vi "PXI-Set AO Gains and Multipliers.vi"(0 "Multipliers":dbl[](array[numeric]), 5 "Gains":dbl[](array[numeric]), 7 "AO Channels":i32[](array[numeric]), 11 "error in (no error)":errorcluster) -> (15 "error out":errorcluster)   [LabVIEW 2020]
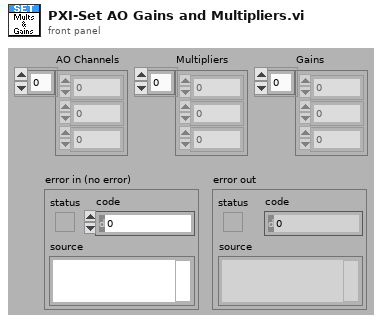
[diagram p1: front panel]
types:
  T1 = enum16{"Init", "Write", "Read", "Latch setup", "Compute comp."}
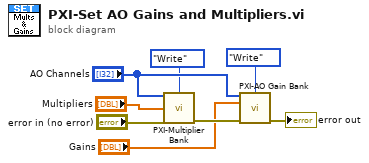
[diagram p0: block diagram]
diagram:
  n1 = call "PXI-Multiplier Bank.vi"("AO Channels"="AO Channels", "Action"=enum16{"Init", "Write", "Read"}."Write", "Multipliers"="Multipliers", "error in (no error)"="error in (no error)") -> ("error out"=w8:errorcluster)  [unwired: 9 in, 2 out]
  n2 = call "PXI-AO Gain Bank.vi"("AO Channels"="AO Channels", "Action"=T1."Write", "Gains"="Gains", "error in (no error)"=w8) -> ("error out"=→"error out":errorcluster)  [unwired: 6 in, 5 out]
